vi "Sound Spectrogram Simple.vi"() -> ()   [LabVIEW 2016]
doc: "This VI illustrates how to perform simultaneous sound IO, i.e., how to continuously play the sound acquired from a microphone. It requires the use of a microphone attached to the sound card. You can specify the IDs of the input and output devices, the frequency to sample at, and the buffer size for both devices. Higher frequencies have better quality, but demand more resources and are limited by the capabilities of your sound card. A large number of samples decreases the risk of glitches, but increases the delay between acquisition and playback."
uses:
  <vilib>/Analysis/4window.llb/windowTd.ctl
  Spectrogram States.ctl
  <vilib>/sound2/lvsound2.llb/Sampling Mode.ctl
  <vilib>/measure/maspectr.llb/Power Spectrum and PSD Export Mode.ctl
  <vilib>/sound2/lvsound2.llb/Sound Input Task ID.ctl
  <vilib>/sound2/lvsound2.llb/Sound Input Read (DBL).vi
  <vilib>/measure/maspectr.llb/FFT Power Spectrum and PSD for N Chan.vi
  <vilib>/measure/NI_MAPro.lvlib
  <vilib>/Analysis/NI_AALPro.lvlib
panel:
  in  "Tab Control":enum32{"Signal", "Settings"}(tab)
  out "Sound Spectrogram":dbl[][](graph)
  out "Acquired Sound":waveform(dbl)[](graph)=[{"t0"=timestamp(3602675551.8619905 s since 1904-01-01), "dt"=2.2675736961451248e-05, "Y"=array[8820 elements]}, {"t0"=timestamp(3602675551.8619905 s since 1904-01-01), "dt"=2.2675736961451248e-05, "Y"=array[8820 elements]}]
  out "Power Spectral Density":cluster{"f0":dbl, "df":dbl, "magnitude":dbl[]}[](graph)
  in  "Sampling":T1={"Rate [S/s]"=44100.0, "Channels"=2.0, "Resolution [Bits]"=16.0} {"Rate [S/s]" format="%#_6p"}
  in  "Interval [s]":dbl=0.2 min=0.1 max=5.0 step=0.1
  in  "Window":T2=1 items=["Rectangle"=0, "Hanning"=1, "Hamming"=2, "Blackman-Harris"=3, "Exact Blackman"=4, "Blackman"=5, "Flat Top"=6, "4 Term B-Harris "=7, "7 Term B-Harris"=8, "Low Sidelobe"=9, "Blackman Nuttall"=11, "Triangle"=30, "Bartlett-Hanning"=31, "Bohman"=32, "Parzen"=33, "Welch"=34, "Kaiser"=60, "Dolph-Chebyshev"=61, "Gaussian"=62]
  in  "Sound Input Device ID":u32
  in  "Stop":bool
  # "Record sound from the computer input device.\nPlot the recorded signal in the time domain, and its power spectrum."
  # "Sound Signal and Frequency Spectrum"
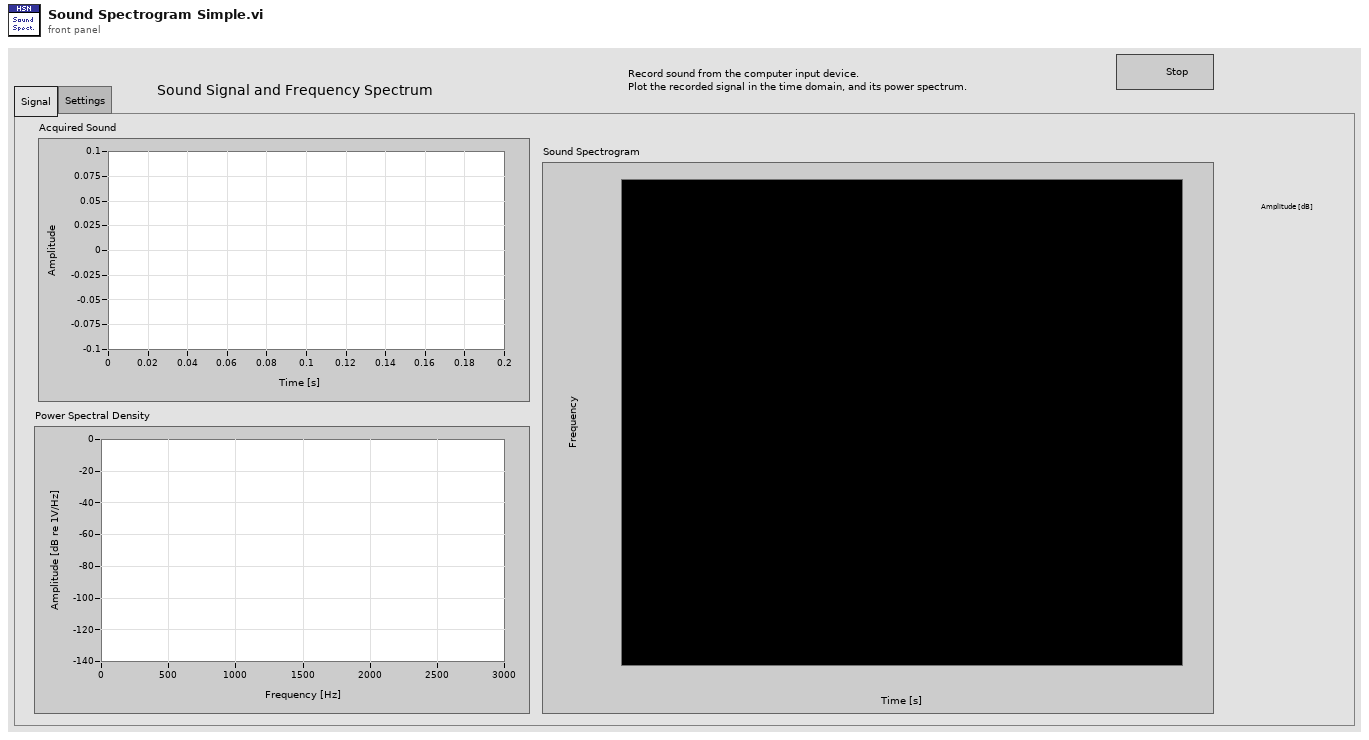
[diagram p1: front panel]
types:
  T1 = cluster{"Rate [S/s]":dbl, "Channels":dbl, "Resolution [Bits]":dbl}
  T2 = typedef "NI_AALPro.lvlib/windowTd.ctl" = u32
  T3 = typedef "Spectrogram States.ctl" = enum16{"Initialize", "Idle", "Acquire", "Process", "Display", "Rescale", "Shutdown", "Quit"}
  T4 = typedef "Sound Input Task ID.ctl" = u32
  T5 = typedef "Sampling Mode.ctl" = i32
  T6 = typedef "NI_MAPro.lvlib/Power Spectrum and PSD Export Mode.ctl" = u16
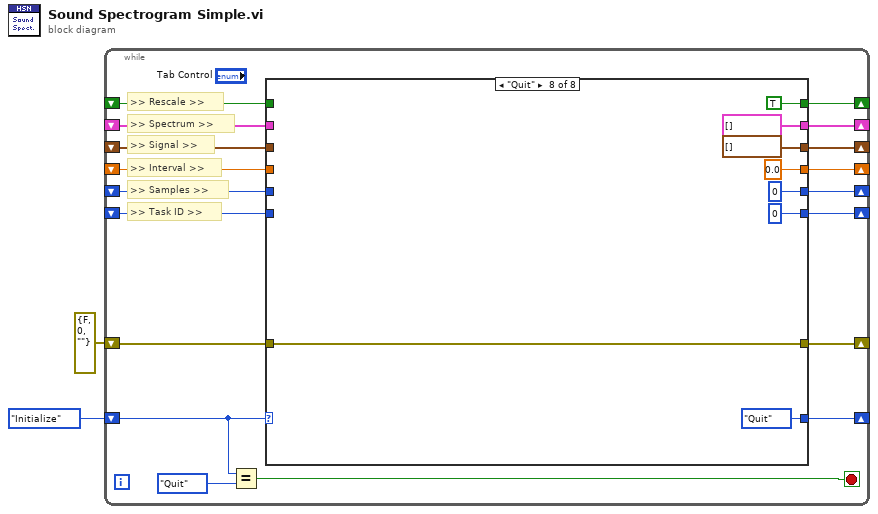
[diagram p0: block diagram]
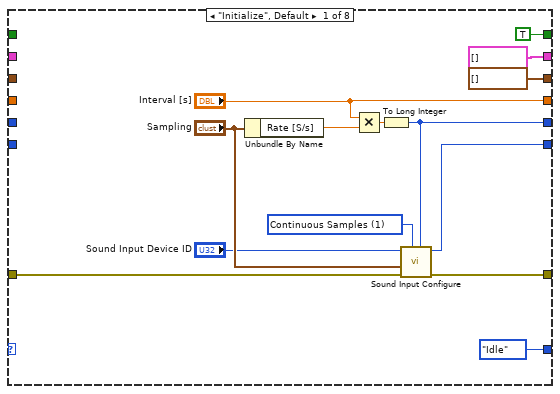
[diagram p2: hidden frame]
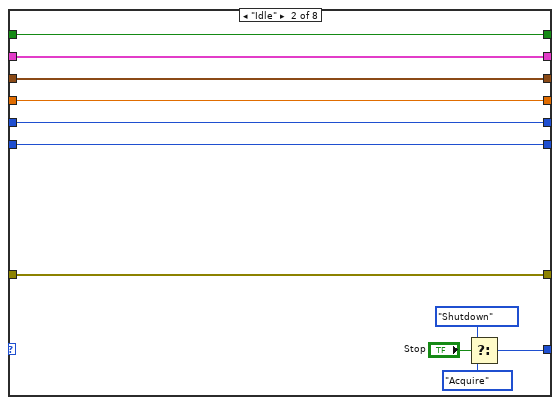
[diagram p3: hidden frame]
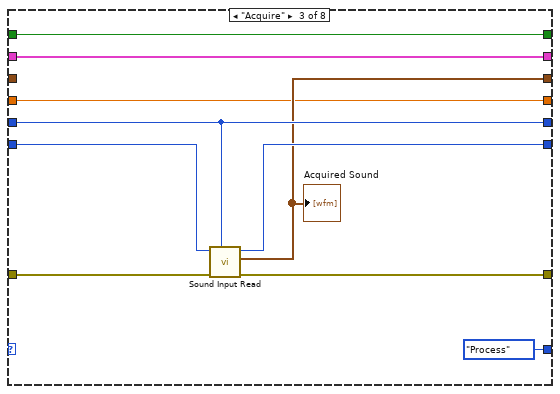
[diagram p4: hidden frame]
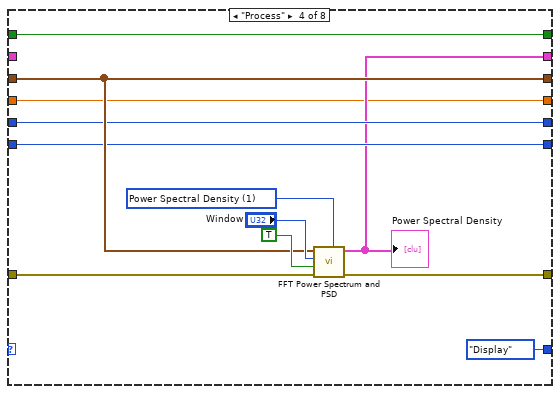
[diagram p5: hidden frame]
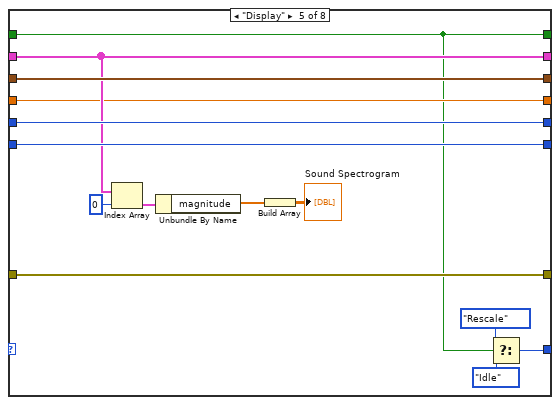
[diagram p6: hidden frame]
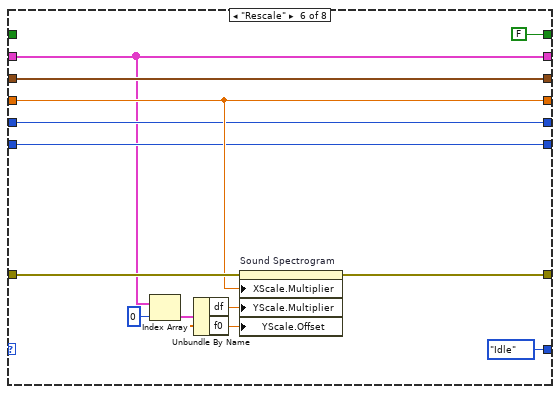
[diagram p7: hidden frame]
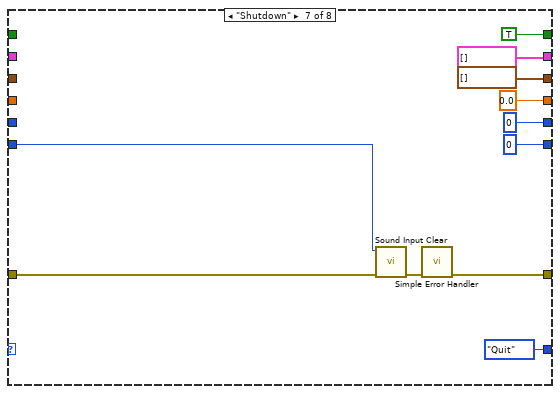
[diagram p8: hidden frame]
diagram:
  n1 = while {
    shift-right: [w20] -> _
    shift-left: errorcluster {"status"=FALSE, "code"=0, "source"=""} ("error out") -> [w19]
    shift-right: [w18] -> _
    shift-left: _ -> [w17]
    shift-right: [w16] -> _
    shift-left: _ -> [w15]
    shift-right: [w14] -> _
    shift-left: Spectrogram_States."Initialize" ("State") -> [w11]
    shift-right: [w13] -> _
    shift-left: _ -> [w12]
    shift-right: [w8] -> _
    shift-left: _ -> [w7]
    shift-right: [w6] -> _
    shift-left: _ -> [w5]
    shift-right: [w4] -> _
    shift-left: _ -> [w3]
    stop <- w9 stop-if-true
    # ">> Spectrum >>"
    # ">> Rescale >>"
    # ">> Interval >>"
    # ">> Signal >>"
    # ">> Task ID >>"
    # ">> Samples >>"
    n2 = Equal?(x=w11, y=Spectrogram_States."Quit") -> (x = y?=w9:bool)
    n3 = case shown="\"Quit\"" w11 {
      tunnel: [w29 w43 w51 w63 w72 w85 w103 w110] -> w20
      tunnel: w19 -> [w28 w43 w52 w64 w72 w93 w105 w110]
      tunnel: [w27 w45 w53 w60 w81 w89 0 0] -> w18
      tunnel: w17 -> [_ w45 w53 w60 w81 w89 _ _]
      tunnel: [w26 w44 w54 w61 w80 w88 T4 0 ("task ID out") T4 0 ("task ID out")] -> w16
      tunnel: w15 -> [_ w44 w55 w61 w80 w88 w101 _]
      tunnel: [Spectrogram_States."Idle" ("State") w39 Spectrogram_States."Process" ("State") Spectrogram_States."Display" ("State") w68 Spectrogram_States."Idle" ("State") Spectrogram_States."Quit" ("State") Spectrogram_States."Quit" ("State")] -> w14
      tunnel: [waveform(dbl)[] [] ("data") w38 w49 w62 w79 w87 waveform(dbl)[] [] ("data") waveform(dbl)[] [] ("data")] -> w13
      tunnel: w12 -> [_ w38 _ w62 w79 w87 _ _]
      tunnel: [cluster{"f0":dbl, "df":dbl, "magnitude":dbl[]}[] [] ("Power Spectrum / PSD") w37 w48 w58 w74 w86 cluster{"f0":dbl, "df":dbl, "magnitude":dbl[]}[] [] ("Power Spectrum / PSD") cluster{"f0":dbl, "df":dbl, "magnitude":dbl[]}[] [] ("Power Spectrum / PSD")] -> w8
      tunnel: w7 -> [_ w37 w48 _ w74 w86 _ _]
      tunnel: ["Interval [s]" w36 w47 w57 w73 w90 0.0 ("Block Size [s]") 0.0 ("Block Size [s]")] -> w6
      tunnel: w5 -> [_ w36 w47 w57 w73 w90 _ _]
      tunnel: [TRUE w35 w46 w56 w71 FALSE TRUE TRUE] -> w4
      tunnel: w3 -> [_ w35 w46 w56 w71 _ _ _]
      frame "Initialize", Default {
        w31 = T5 1 items=["Finite Samples", "Continuous Samples"] ("sample mode")
        n4 = Unbundle By Name("Sampling") -> ("Rate [S/s]"=w33:dbl)
        n5 = Multiply(x="Interval [s]", y=w33) -> (x*y=w34:dbl)
        n6 = To Long Integer(number=w34) -> (32bit integer=w27:i32)
        n7 = call <vilib>:"Sound Input Configure.vi"("number of samples/ch"=w27, "sample mode"=w31, "error in (no error)"=w28, "sound format"="Sampling", "device ID"="Sound Input Device ID") -> ("error out"=w29:errorcluster, "task ID"=w26:T4)  [unwired: 5 in]
      }
      frame "Idle" {
        n8 = Select(t=Spectrogram_States."Shutdown" ("State"), s="Stop", f=Spectrogram_States."Acquire" ("State")) -> (s? t:f=w39:T3)
      }
      frame "Acquire" {
        n9 = call-poly <vilib>:"Sound Input Read.vi"("number of samples/ch"=w53, "error in (no error)"=w52, "task ID"=w55) -> ("error out"=w51:errorcluster, "data"=w49:waveform(dbl)[], "task ID out"=w54:T4)  [unwired: 6 in]
        "Acquired Sound" <- w49
      }
      frame "Process" {
        w67 = T6 1 items=["Power Spectrum", "Power Spectral Density"] ("export mode")
        n10 = call-poly <vilib>:"FFT Power Spectrum and PSD.vi"("export mode"=w67, "error in (no error)"=w64, "dB On (F)"=TRUE, "window"="Window", "time signals"=w62) -> ("error out"=w63:errorcluster, "Power Spectrum / PSD"=w58:cluster{"f0":dbl, "df":dbl, "magnitude":dbl[]}[])  [unwired: 3 in, 2 out]
        "Power Spectral Density" <- w58
      }
      frame "Display" {
        n11 = Index Array(array=w74, index=0) -> (element=w78:cluster{"f0":dbl, "df":dbl, "magnitude":dbl[]})
        n12 = Unbundle By Name(w78) -> ("magnitude"=w76:dbl[])
        n13 = Build Array(w76) -> (→"Sound Spectrogram":dbl[][])
        n14 = Select(t=Spectrogram_States."Rescale" ("State"), s=w71, f=Spectrogram_States."Idle" ("State")) -> (s? t:f=w68:T3)
      }
      frame "Rescale" {
        n15 = Index Array(array=w86, index=0) -> (element=w94:cluster{"f0":dbl, "df":dbl, "magnitude":dbl[]})
        n16 = Unbundle By Name(w94) -> ("df"=w91:dbl, "f0"=w92:dbl)
        n17 = property on="Sound Spectrogram" class="IntChart (strict)"(error in=w93, "XScale.Multiplier"=w90, "YScale.Multiplier"=w91, "YScale.Offset"=w92) -> (error out=w85:errorcluster)  [unwired: 1 in, 1 out]
      }
      frame "Shutdown" {
        n18 = call <vilib>:"Sound Input Clear.vi"("error in (no error)"=w105, "task ID"=w101) -> ("error out"=w104:errorcluster)  [unwired: 9 in]
        n19 = call <vilib>:"Simple Error Handler.vi"("error in (no error)"=w104) -> ("error out"=w103:errorcluster)  [unwired: 4 in, 4 out]
      }
      frame "Quit" {
      }
    }
  }
